vi "GenerateSyntheticRI.vi"(0 "Number of Wavelengths WL":dbl) -> (1 "Real Part per WL":dbl[](array[numeric]), 2 "Imaginary Part per WL":dbl[](array[numeric]), 3 "RealUncertainty":dbl[](array[numeric]), 4 "ImagiUncertainty":dbl[](array[numeric]))   [LabVIEW 2013]
uses:
  <vilib>/imath/engines/lvmath2/RunTimeEngine/ErrorHandling/NIMS_Finalize Error.vi
  <vilib>/imath/engines/lvmath2/RunTimeEngine/NodeEndStatement/NIMS_NodeEndStatement_Output.vi
  <instcachedir>/0/NIMS_NodeEndStatement_Output_53EC0D466D134D7ABD903AC30B43404B.lvgen/NIMS_NodeEndStatement_Output_53EC0D466D134D7ABD903AC30B43404B_005.vi
  <vilib>/imath/engines/lvmath2/RunTimeEngine/RangeToken/NIMS_Range.vi
  <instcachedir>/0/NIMS_Range_7481B155BEE341ECA0F59DDB444E2C09.lvgen/NIMS_Range_7481B155BEE341ECA0F59DDB444E2C09_000.vi
  <vilib>/imathl/engines/lvmath/Functions/Error Handling/Create Error.vi
  <vilib>/imath/engines/lvmath2/RunTimeEngine/ArithmeticOperatorToken/NIMS_ArithmeticOperator_times.vi
  <instcachedir>/0/NIMS_ArithmeticOperator_times_F6527734CE75451889337B8CE94765C6.lvgen/NIMS_ArithmeticOperator_times_F6527734CE75451889337B8CE94765C6_000.vi
  <vilib>/imath/engines/lvmath2/RunTimeEngine/BuiltInFunctions/abs/NIMS_abs(signed).vi
  <instcachedir>/0/NIMS_abs(signed)_C4FCB8E6058B49B797C7C8D53CA5F6EC.lvgen/NIMS_abs(signed)_C4FCB8E6058B49B797C7C8D53CA5F6EC_001.vi
panel:
  out "size(s)":i32
  out "RI Graph":T1(graph)=[{"Ramp Pattern"=[1.7709090992870622, 2.2136363741088276, 2.656363648930593, 3.0990909237523585, 3.5418181985741244, 3.98454547339589, 4.427272748217655], "Extinction"=[2.6163673e-09, 3.3294045e-09, 4.1920147e-09, 4.6714708e-09, 6.2441643e-09, 8.2969445e-09, 9.5108899e-09]}, {"Ramp Pattern"=array[1000 elements], "Extinction"=array[1000 elements]}]
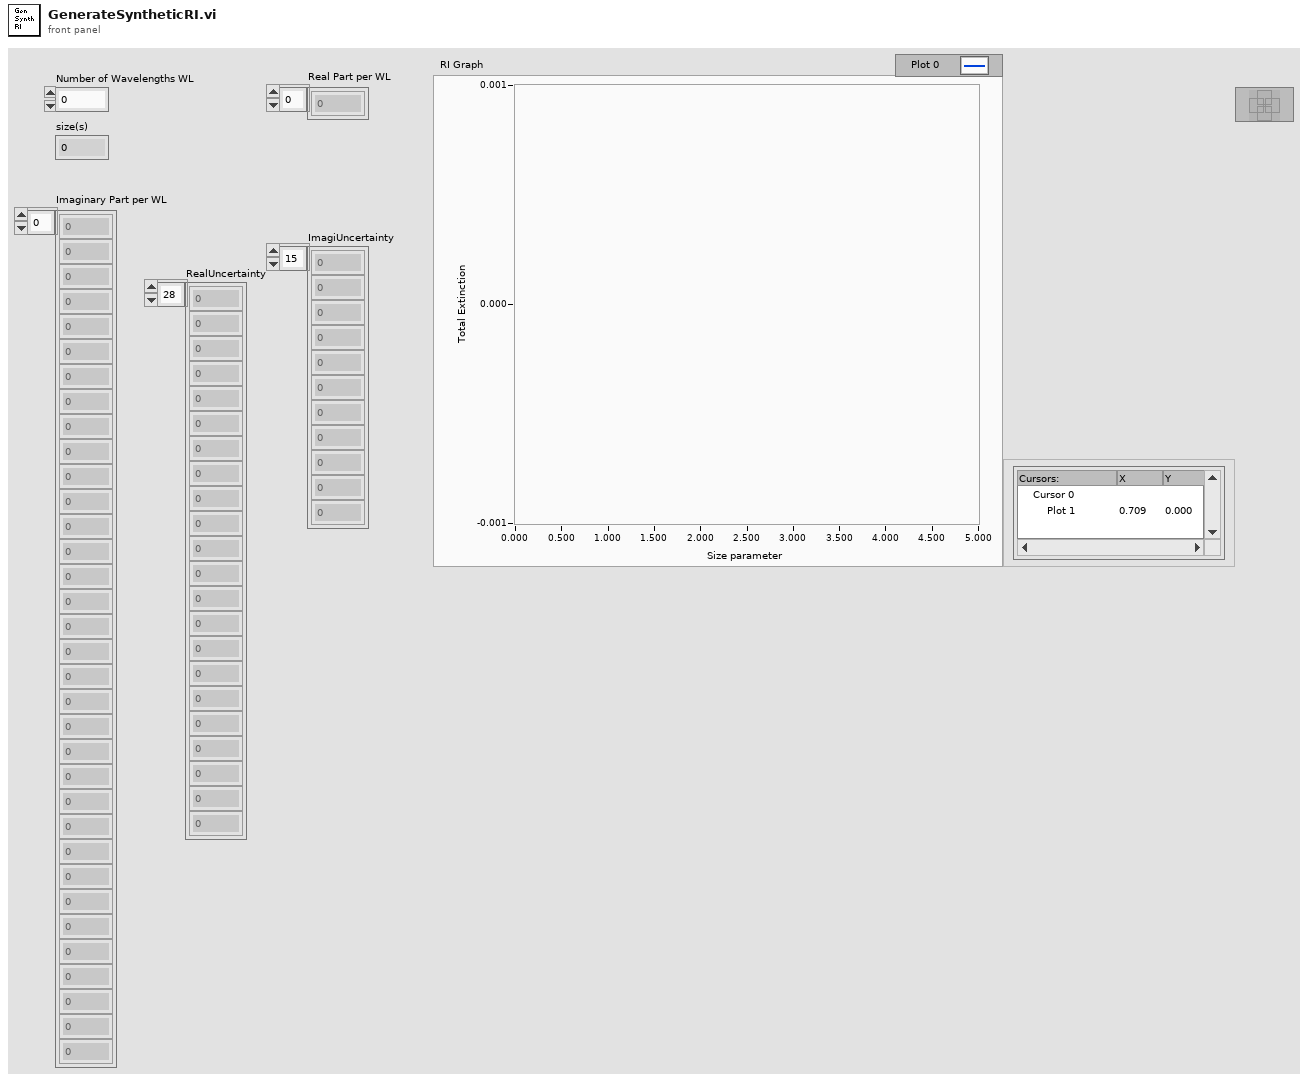
[diagram p1: front panel]
types:
  T1 = cluster{"Ramp Pattern":dbl[], "Extinction":dbl[]}[]
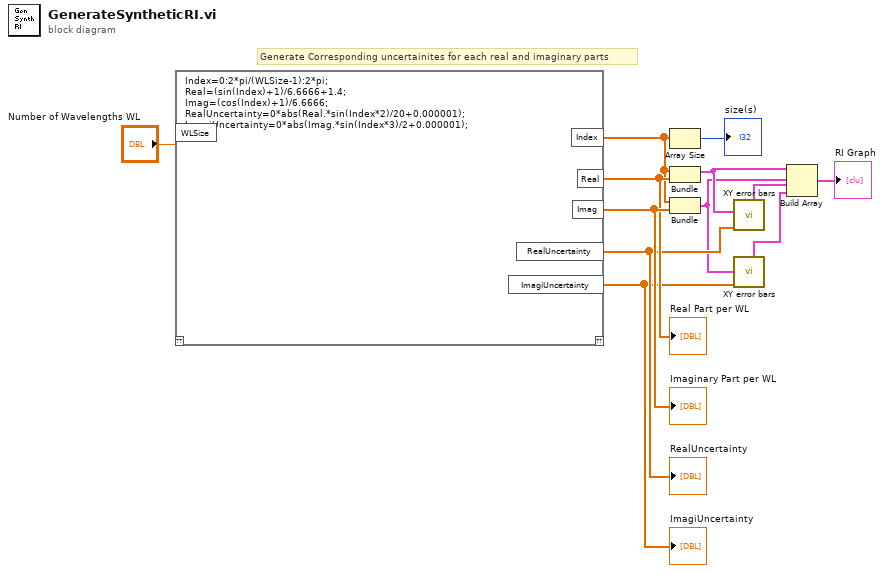
[diagram p0: block diagram]
diagram:
  # "Generate Corresponding uncertainites for each real and imaginary parts"
  n1 = mathscript code="Index=0:2*pi/(WLSize-1):2*pi;\nReal=(sin(Index)+1)/6.6666+1.4;\nImag=(cos(Index)+1)/6.6666;\nRealUncertainty=0*abs(Real.*sin(Index*2)/20+0.000001);\nImagiUncertainty=0*abs(Imag.*sin(Index*3)/2+0.000001);"("WLSize"="Number of Wavelengths WL") -> ("Index"=w8:dbl[], "Real"=w9:dbl[], "Imag"=w11:dbl[], "RealUncertainty"=w5:dbl[], "ImagiUncertainty"=w2:dbl[])  [unwired: 1 in, 1 out]
  "Real Part per WL" <- w9
  "Imaginary Part per WL" <- w11
  "RealUncertainty" <- w5
  "ImagiUncertainty" <- w2
  n2 = Array Size(array=w8) -> (size(s)=→"size(s)":i32)
  n3 = Bundle("Index"=w8, "Real"=w9) -> (w6:cluster{"Index":dbl[], "Real":dbl[]})  [unwired: 1 in]
  n4 = Bundle("Index"=w8, "Imag"=w11) -> (w3:cluster{"Index":dbl[], "Imag":dbl[]})  [unwired: 1 in]
  n5 = call "XY error bars.vi"("XY plot"=w6, "Yerror"=w5) -> ("Y error bars"=w4:cluster{dbl[], dbl[]})  [unwired: 6 in, 2 out]
  n6 = call "XY error bars.vi"("XY plot"=w3, "Yerror"=w2) -> ("Y error bars"=w1:cluster{dbl[], dbl[]})  [unwired: 6 in, 2 out]
  n7 = Build Array(w6, w3, w4, w1) -> (→"RI Graph":cluster{"Index":dbl[], "Imag":dbl[]}[])
